vi "FH 55.vi"() -> ()   [LabVIEW 2014, in "FH 55.lvlib"]
uses:
  FH 55.lvlib
  TypeDef/VisaCluster.ctl
  TypeDef/command.ctl
  TypeDef/Unit.ctl
  TypeDef/Range.ctl
  TypeDef/Temp_Unit.ctl
  TypeDef/Max.ctl
  TypeDef/Unit2.ctl
  TypeDef/Display.ctl
  TypeDef/Value_String.ctl
panel:
  in  "Control":T6 {"Lower"."Numeric" format="%#_4f"; "Set_Rel"."Numeric" format="%#_4f"; "UPPER"."Numeric" format="%#_4f"}
  in  "Array":string[](array[string])
  out "measured values":string
  in  "measured values":cluster{"Numeric":i32, "OK Button":bool}
  out "FH 55 Gauss-/Teslameter":T7
  in  "Stop":bool
  in  "OK":bool
  out "Busy":bool
  in  "Cluster":T8
  in  "Init":bool
  in  "Local":bool
  in  "Reset":bool
  in  "Zero":bool
  out "time current":u32
  out "loop 2":i32
  out "loop 1":i32
  out "error out":errorcluster
  in  "error in (no error)":errorcluster
  out "VisaCluster":T9
  in  "VisaCluster":T9={"VISA Resource Name"="COM1"}
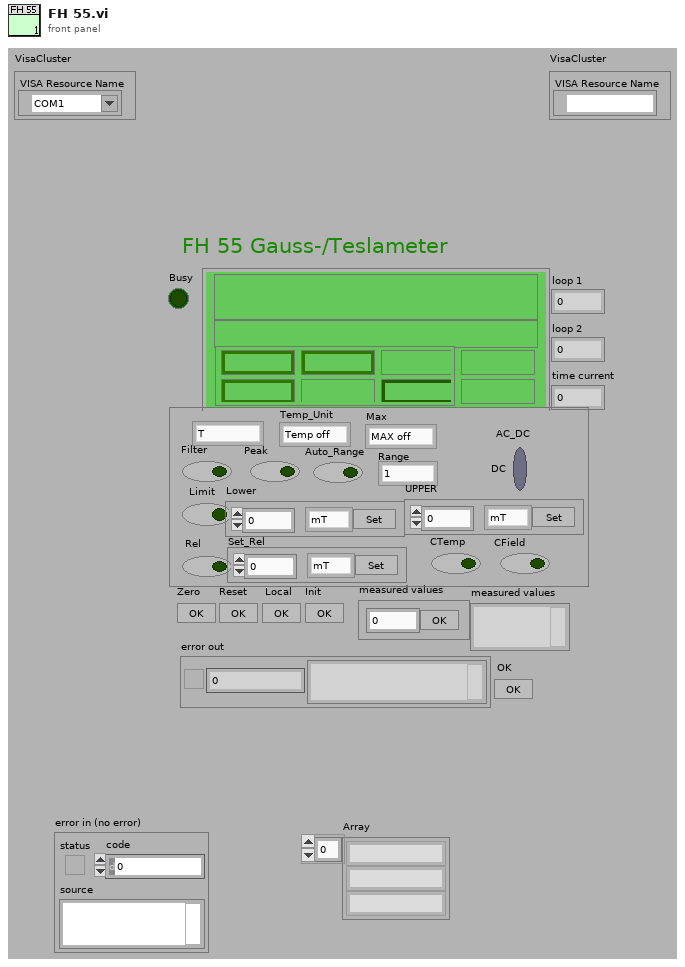
[diagram p1: front panel]
types:
  T1 = typedef "FH 55.lvlib/Range.ctl" = enum16{"1", "2", "3", "4", "5", "6", "7"}
  T2 = typedef "FH 55.lvlib/Unit2.ctl" = enum16{"mT", "G", "kA/m"}
  T3 = typedef "FH 55.lvlib/Unit.ctl" = enum16{"T", "G", "A/m"}
  T4 = typedef "FH 55.lvlib/Temp_Unit.ctl" = enum16{"Temp off", "Celsius", "Fahrenheit"}
  T5 = typedef "FH 55.lvlib/Max.ctl" = enum16{"MAX off", "Show MAX", "MAX/MIN"}
  T6 = cluster{" Peak":bool, " Limit":bool, " Filter":bool, " Auto_Range":bool, " Rel":bool, "AC_DC ":bool, "Range":T1, " CField":bool, " CTemp":bool, "UPPER":cluster{"Numeric":dbl, "Cancel Button":bool, "Unit":T2}, "Set_Rel":cluster{"Numeric":dbl, "Cancel Button":bool, "Unit":T2}, "Unit":T3, "Temp_Unit":T4, "Max":T5, "Lower":cluster{"Numeric":dbl, "Cancel Button":bool, "Unit":T2}}
  T7 = typedef "FH 55.lvlib/Display.ctl" = cluster{"current value":string, "Limit":string, "Remote":string, "function ":string, "Cluster":cluster{"AC/DC":string, "Auto":string, "Filter":string, "Range":string, "Rel":string, "Peak":string}}
  T8 = typedef "FH 55.lvlib/command.ctl" = cluster{"String":string, "Boolean":bool, "Unit":T3, "Range":T1, "Temp_Unit":T4, "Max":T5, "Numeric":i32, "Set_lower":cluster{"Numeric":i64, "Cancel Button":bool, "Unit":T2}}
  T9 = typedef "FH 55.lvlib/VisaCluster.ctl" = cluster{"VISA Resource Name":refnum<visa-resource-name>}
  T10 = cluster{"Peak":bool, "Limit":bool, "Filter":bool, "Auto_Range":bool, "Rel":bool, "AC_DC":bool, "Range":T1, "CField":bool, "CTemp":bool, "UPPER":cluster{"Numeric":dbl, "Cancel Button":bool, "Unit":T2}, "Set_Rel":cluster{"Numeric":dbl, "Cancel Button":bool, "Unit":T2}, "Unit":T3, "Temp_Unit":T4, "Max":T5, "Lower":cluster{"Numeric":dbl, "Cancel Button":bool, "Unit":T2}}
  T11 = typedef "FH 55.lvlib/Value_String.ctl" = cluster{"Numeric":dbl, "String":string}
  T12 = cluster{"current value":string, "Temperature":string, "Limit":string, "function":string, "Cluster":cluster{"AC/DC":string, "Auto":string, "Filter":string, "Range":string, "Rel":string, "Peak":string}}
  T13 = cluster{"AC/DC":string, "Auto":string, "Filter":string, "Range":string, "Rel":string, "Peak":string}
  T14 = typedef "Semaphore RefNum" = refnum<k1>
  T15 = cluster{"Numeric":i64, "Cancel Button":bool, "Unit":T2}
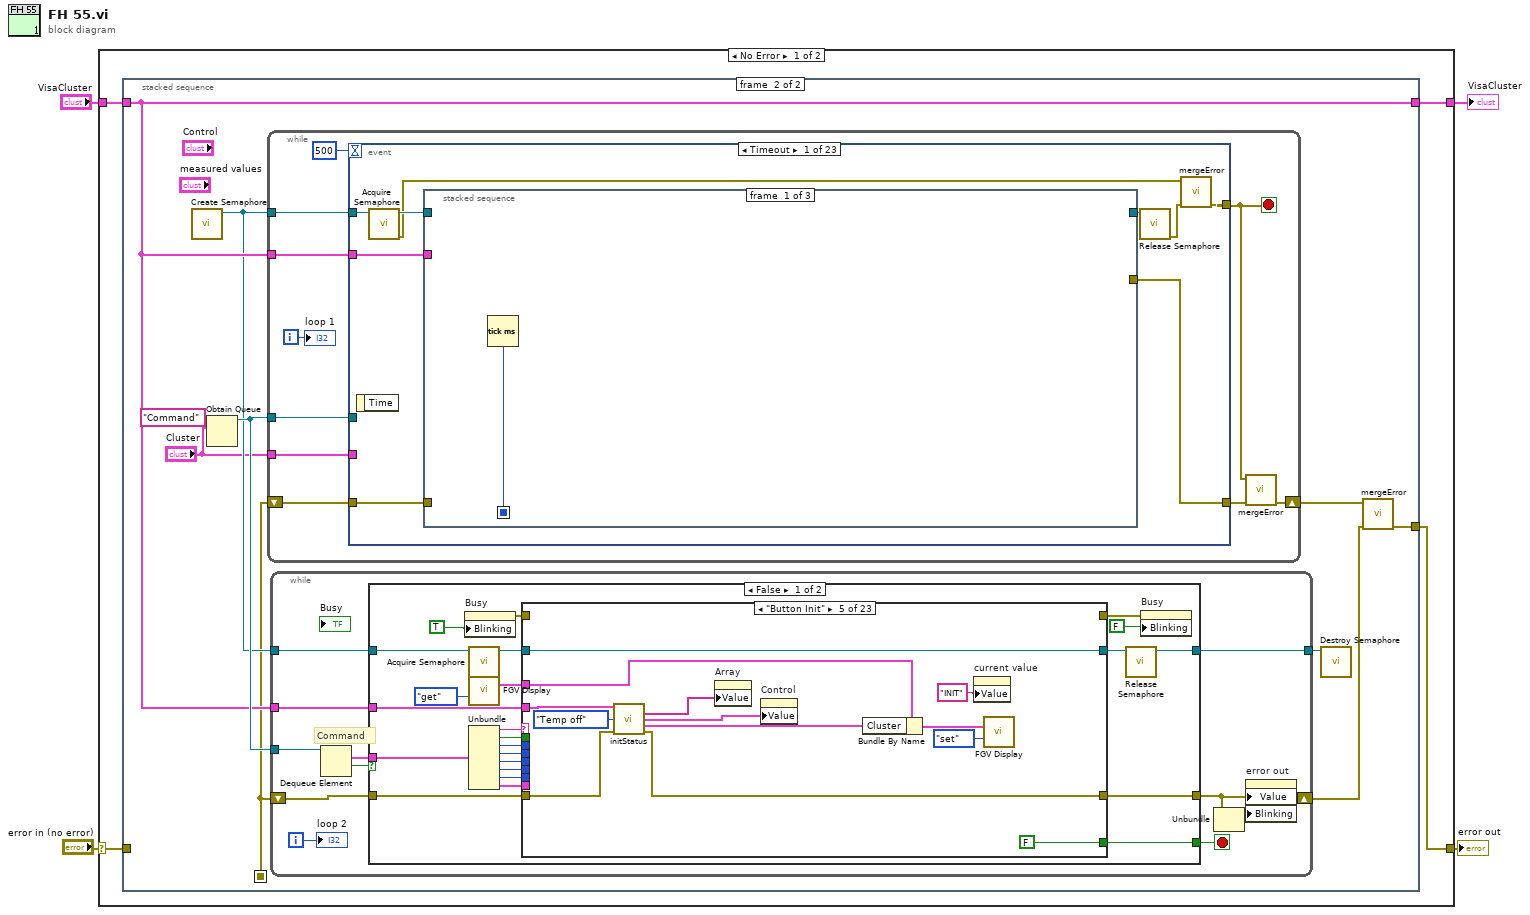
[diagram p0: block diagram]
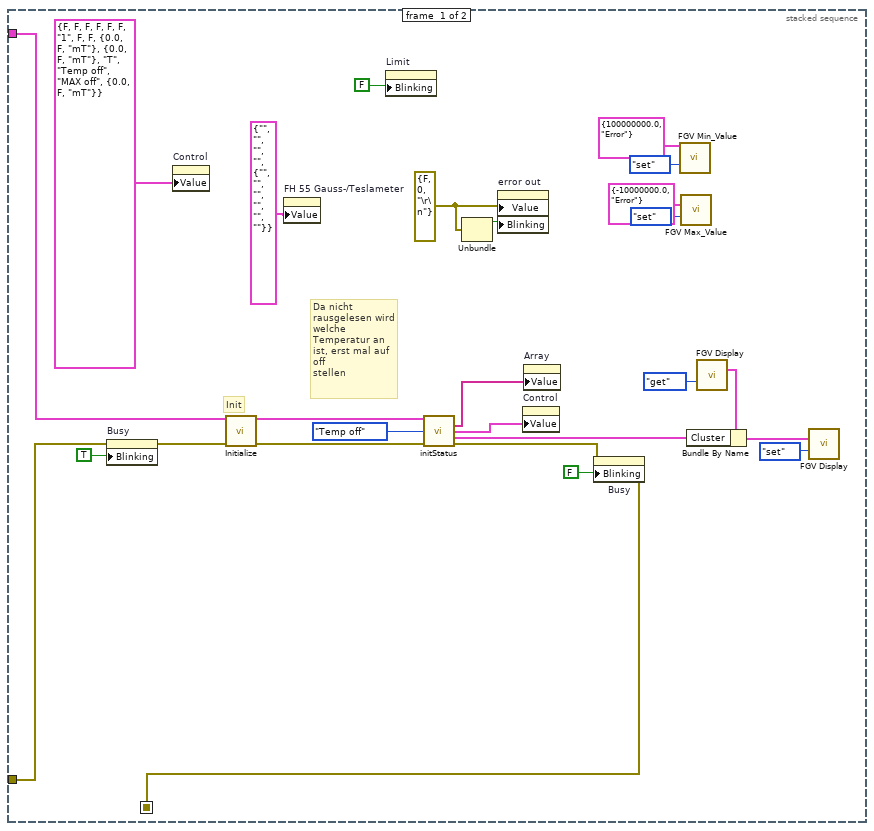
[diagram p2: hidden frame]
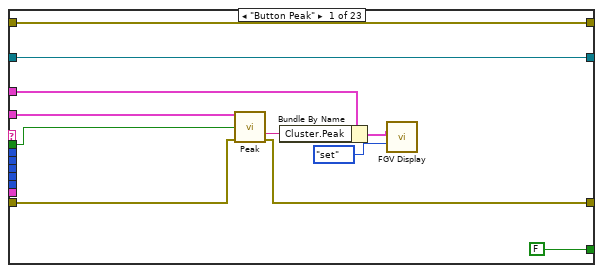
[diagram p3: hidden frame]
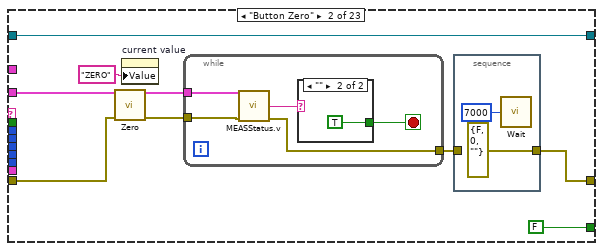
[diagram p4: hidden frame]
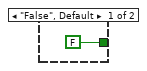
[diagram p5: hidden frame]
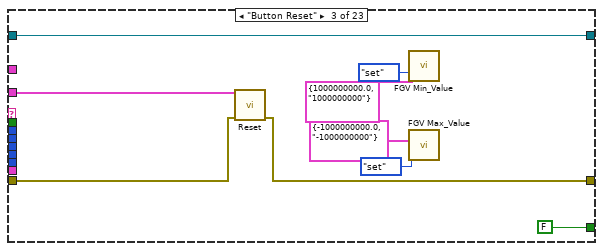
[diagram p6: hidden frame]
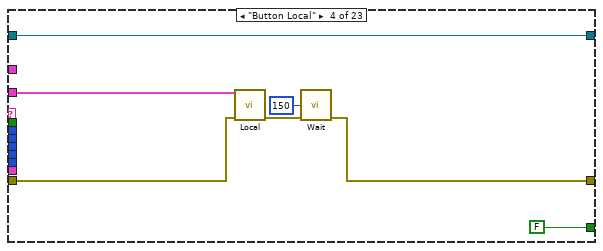
[diagram p7: hidden frame]
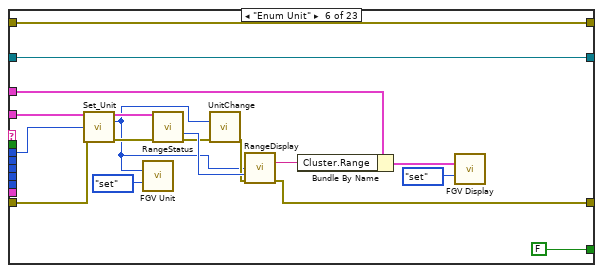
[diagram p8: hidden frame]
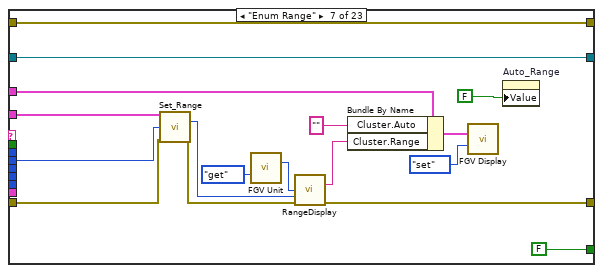
[diagram p9: hidden frame]
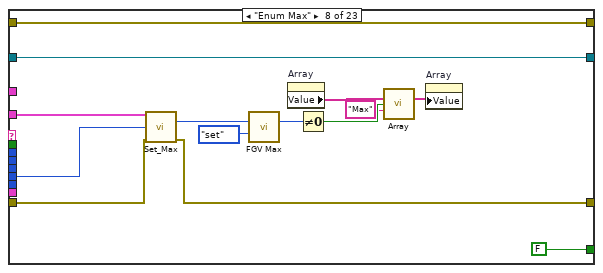
[diagram p10: hidden frame]
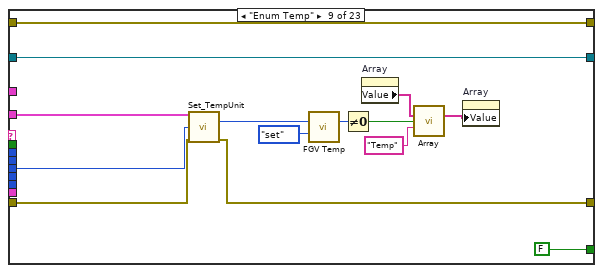
[diagram p11: hidden frame]
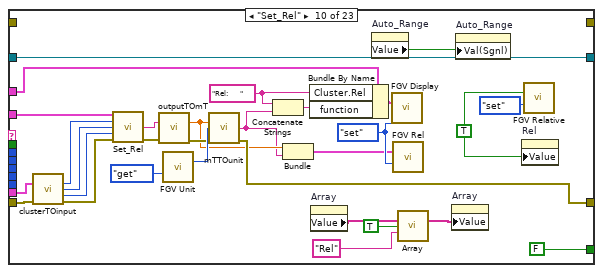
[diagram p12: hidden frame]
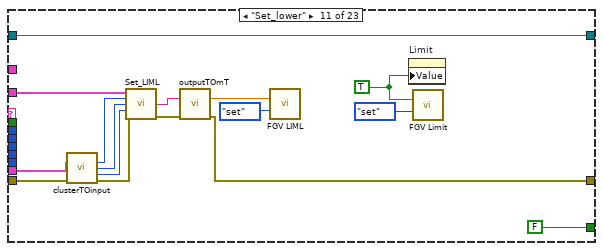
[diagram p13: hidden frame]
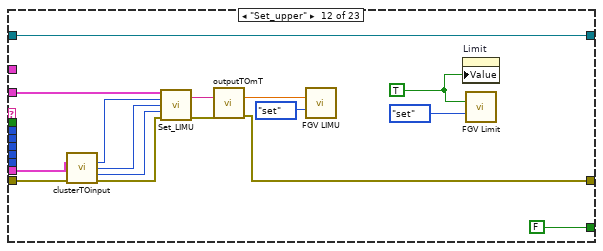
[diagram p14: hidden frame]
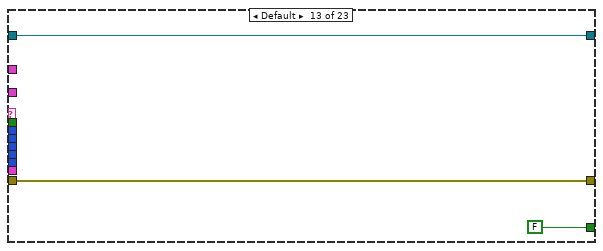
[diagram p15: hidden frame]
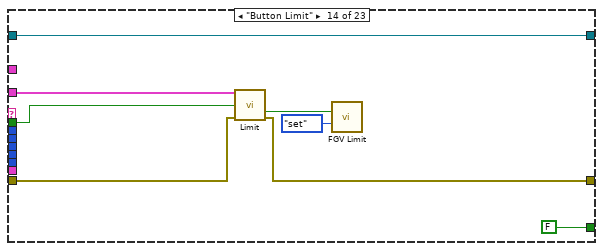
[diagram p16: hidden frame]
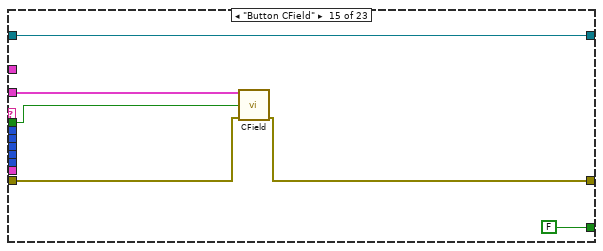
[diagram p17: hidden frame]
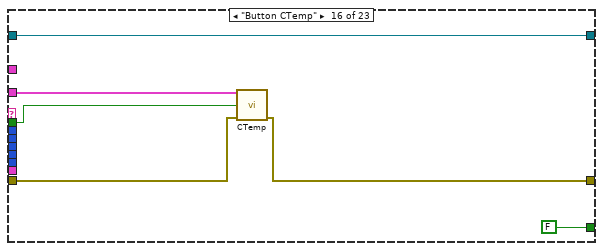
[diagram p18: hidden frame]
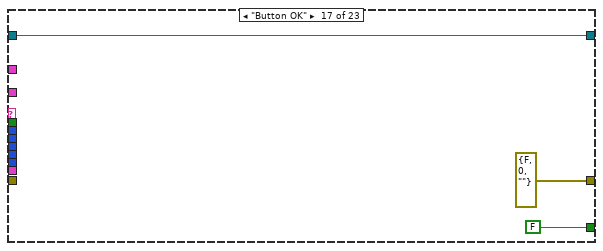
[diagram p19: hidden frame]
diagram:
  n1 = case shown="No Error" "error in (no error)" {
    selector: "error in (no error)" -> [w7 w591]
    tunnel: "VisaCluster" -> [w8 w592]
    tunnel: [w6 w592] -> w3
    tunnel: [w5 w591] -> w1
    frame No Error {
      n2 = stacked-sequence {
        seq-local: [w13 _] -> [_ w35]
        tunnel: w8 -> [w34 w42]
        tunnel: w7 -> [w22 _]
        tunnel: [_ w42] -> w6
        tunnel: [_ w39] -> w5
        frame #0 {
          w16 = errorcluster {"status"=FALSE, "code"=0, "source"="\r\n"} ("error out")
          # "Init"
          # "Da nicht rausgelesen wird welche \nTemperatur an ist, erst mal auf off \nstellen"
          n3 = property on="Busy" class="Bool (strict)"(error in=w22, "Blinking"=TRUE) -> (error out=w21:errorcluster)  [unwired: 1 in, 1 out]
          n4 = property on="Control" class="Clust (strict)"("Value"=T10 {"Peak"=FALSE, "Limit"=FALSE, "Filter"=FALSE, "Auto_Range"=FALSE, "Rel"=FALSE, "AC_DC"=FALSE, "Range"=enum."1", "CField"=FALSE, "CTemp"=FALSE, "UPPER"={"Numeric"=0.0, "Cancel Button"=FALSE, "Unit"=enum."mT"}, "Set_Rel"={"Numeric"=0.0, "Cancel Button"=FALSE, "Unit"=enum."mT"}, "Unit"=enum."T", "Temp_Unit"=enum."Temp off", "Max"=enum."MAX off", "Lower"={"Numeric"=0.0, "Cancel Button"=FALSE, "Unit"=enum."mT"}} ("Control")) -> ()  [unwired: 2 in, 2 out]
          n5 = call "Initialize.vi"("VisaCluster"=w34, "error in (no error)"=w21) -> ("VisaCluster"=w31:T9, "error out"=w30:errorcluster)  [unwired: 12 in]
          n6 = property on="FH 55 Gauss-/Teslameter" class="Clust (strict)"("Value"=T12 {"current value"="", "Temperature"="", "Limit"="", "function"="", "Cluster"={"AC/DC"="", "Auto"="", "Filter"="", "Range"="", "Rel"="", "Peak"=""}}) -> ()  [unwired: 2 in, 2 out]
          n7 = property on="Limit" class="Str"("Blinking"=FALSE) -> ()  [unwired: 2 in, 2 out]
          n8 = call "initStatus.vi"("VisaCluster"=w31, "Temp_Unit"=Temp_Unit."Temp off", "error in (no error)"=w30) -> ("Array"=w9:string[], "Control"=w10:T6, "Display"=w27:T13, "error out"=w24:errorcluster)  [unwired: 8 in, 1 out]
          n9 = Unbundle(w16) -> ("status"=w15:bool)  [unwired: 2 out]
          n10 = property on="error out" class="Clust (strict)"("Value"=w16, "Blinking"=w15) -> ()  [unwired: 2 in, 2 out]
          n11 = property on="Control" class="Clust (strict)"("Value"=w10) -> ()  [unwired: 2 in, 2 out]
          n12 = property on="Array" class="Arr (strict)"("Value"=w9) -> ()  [unwired: 2 in, 2 out]
          n13 = property on="Busy" class="Bool (strict)"(error in=w24, "Blinking"=FALSE) -> (error out=w13:errorcluster)  [unwired: 1 in, 1 out]
          n14 = call "FGV Min_Value.vi"("Extrem_Value"=T11 {"Numeric"=100000000.0, "String"="Error"}, "action"=enum16{"set", "get"}."set") -> ()  [unwired: 13 in, 1 out]
          n15 = call "FGV Max_Value.vi"("Extrem_Value"=T11 {"Numeric"=-10000000.0, "String"="Error"}, "action"=enum16{"set", "get"}."set") -> ()  [unwired: 13 in, 1 out]
          n16 = call "FGV Display.vi"("action"=enum16{"set", "get"}."get") -> ("FH 55 Gauss-/Teslameter 2"=w28:T7)  [unwired: 14 in]
          n17 = Bundle By Name(cluster=w28, "Cluster"=w27) -> (w26:T7)
          n18 = call "FGV Display.vi"("FH 55 Gauss-/Teslameter"=w26, "action"=enum16{"set", "get"}."set") -> ()  [unwired: 13 in, 1 out]
        }
        frame #1 {
          n19 = call <vilib>:"Create Semaphore.vi"() -> ("semaphore"=w41:T14)  [unwired: 5 in, 2 out]
          n20 = Obtain Queue(name (unnamed)="Command", element data type="Cluster") -> (queue out=w43:refnum<queue>)  [unwired: 3 in, 2 out]
          n21 = while {
            tunnel: w42 -> [w378]
            tunnel: w43 -> [w376]
            tunnel: "Cluster" -> [w375]
            tunnel: w41 -> [w374]
            shift-right: [w372] -> w36
            shift-left: w35 -> [w370]
            i -> [w369]
            stop <- w371 stop-if-true
            n22 = event shown="[0] Timeout" {
              selector: _ -> [_ _ _ _ _ _ _ _ _ _ _ _ _ _ _ _ _ _ _ _ _ _ _]
              dyn-events: _ -> [_ _ _ _ _ _ _ _ _ _ _ _ _ _ _ _ _ _ _ _ _ _ _]
              timeout: 500 -> [_ _ _ _ _ _ _ _ _ _ _ _ _ _ _ _ _ _ _ _ _ _ _]
              tunnel: w378 -> [w387 _ _ _ _ _ _ _ _ _ _ _ _ _ _ _ _ _ _ _ _ _ _]
              tunnel: w376 -> [_ w451 w457 w465 w475 w485 w495 w501 w508 w514 w520 w526 w532 w538 w544 w549 w554 w559 w564 w570 w576 w582 w588]
              tunnel: w375 -> [_ w452 w458 w464 w469 w480 w491 w500 w507 w513 w519 w525 w531 w537 w543 w548 w553 w558 w563 w569 w575 w581 w587]
              tunnel: w374 -> [w386 _ _ _ _ _ _ _ _ _ _ _ _ _ _ _ _ _ _ _ _ _ _]
              tunnel: [w382 _ _ _ _ _ _ _ _ _ _ _ _ _ _ _ _ _ _ _ _ _ _] -> w371
              tunnel: [w383 w450 w456 w463 w474 w484 w494 w499 w506 w512 w518 w524 w530 w536 w542 w547 w552 w557 w562 w568 w574 w580 w586] -> w373
              tunnel: w370 -> [w379 w450 w456 w463 w474 w484 w494 w499 w506 w512 w518 w524 w530 w536 w542 w547 w552 w557 w562 w568 w574 w580 w586]
              event Timeout {
                n23 = event-data() -> ()  [unwired: 1 in, 1 out]
                n24 = call <vilib>:"Acquire Semaphore.vi"("semaphore"=w386) -> ("error out"=w380:errorcluster, "semaphore out"=w385:T14)  [unwired: 4 in, 1 out]
                n25 = stacked-sequence {
                  seq-local: [w388 _ _] -> [_ _ w448]
                  tunnel: w387 -> [_ w417 _]
                  tunnel: w385 -> [_ w411 _]
                  tunnel: [_ w411 _] -> w384
                  tunnel: [_ w407 _] -> w383
                  tunnel: w379 -> [_ w404 _]
                  frame #0 {
                    n26 = Tick Count (ms)() -> (millisecond timer value=w388:u32)
                  }
                  frame #1 {
                    w391 = enum16{"set", "get"}."get" ("action")
                    n27 = call "FGV Max.vi"("action"=enum16{"set", "get"}."get") -> ("Max 2"=w400:T5)  [unwired: 14 in]
                    n28 = case shown="\"Show MAX\"" w400 {
                      tunnel: w417 -> [w427 w433 w439]
                      tunnel: [w426 w432 w438] -> w414
                      tunnel: w404 -> [w425 w431 w437]
                      tunnel: [w424 w430 w436] -> w403
                      tunnel: [w423 w429 w435] -> w401
                      frame "Show MAX" {
                        n29 = call "MEASStatus.v.vi"("VisaCluster"=w427, "Time (150) ms"=u32 200, "error in (no error)"=w425) -> ("VisaCluster"=w426:T9, "Answer"=w423:string, "error out"=w424:errorcluster)  [unwired: 10 in]
                      }
                      frame "MAX/MIN" {
                        n30 = call "MEASStatus.v.vi"("VisaCluster"=w433, "Time (150) ms"=u32 200, "error in (no error)"=w431) -> ("VisaCluster"=w432:T9, "Answer"=w429:string, "error out"=w430:errorcluster)  [unwired: 10 in]
                      }
                      frame "MAX off" {
                        n31 = call "MEASStatus.v.vi"("VisaCluster"=w439, "Time (150) ms"=u32 150, "error in (no error)"=w437) -> ("VisaCluster"=w438:T9, "Answer"=w435:string, "error out"=w436:errorcluster)  [unwired: 10 in]
                      }
                    }
                    n32 = call "FGV Limit.vi"("action"=enum16{"set", "get"}."get") -> ("Limit"=w408:bool)  [unwired: 14 in]
                    n33 = call "LimitFunktion.vi"("String"=w401, "Boolean"=w408) -> ("Answer"=w409:string)  [unwired: 12 in, 1 out]
                    n34 = call "MaxFunktion.vi"("VisaCluster"=w414, "Measurment"=w401, "Max"=w400, "error in (no error)"=w403) -> ("VisaCluster 2"=w413:T9, "Answer"=w395:string, "error out"=w402:errorcluster)  [unwired: 8 in, 1 out]
                    n35 = call "FGV Temp.vi"("action"=w391) -> ("Temp_Unit 2"=w412:T4)  [unwired: 14 in]
                    n36 = Index Array(array="Array", index=0) -> (element=w397:string)
                    n37 = case shown="True" w408 {
                      tunnel: w409 -> [_ w444]
                      frame False {
                        n38 = property on="Limit" class="Str"("Blinking"=FALSE) -> ()  [unwired: 2 in, 2 out]
                      }
                      frame True {
                        n39 = case shown="Default" w444 {
                          frame "OK" {
                            n40 = property on="Limit" class="Str"("Blinking"=FALSE) -> ()  [unwired: 2 in, 2 out]
                          }
                          frame Default {
                            n41 = property on="Limit" class="Str"("Blinking"=TRUE) -> ()  [unwired: 2 in, 2 out]
                          }
                        }
                      }
                    }
                    n42 = call "TempDisplay.vi"("VisaCluster"=w413, "Temp_Unit"=w412, "error in (no error)"=w402) -> ("Answer"=w396:string, "error out"=w393:errorcluster)  [unwired: 9 in, 2 out]
                    n43 = call "FGV Relative.vi"("action"=w391) -> ("Rel"=w389:bool)  [unwired: 14 in]
                    n44 = call "RelDisplay.vi"("Boolean"=w389, "error in (no error)"=w393) -> ("Answer"=w390:string, "error out"=w392:errorcluster)  [unwired: 11 in, 1 out]
                    n45 = case shown="Default" w397 {
                      tunnel: w396 -> [_ w419 _ _]
                      tunnel: w395 -> [w418 _ _ _]
                      tunnel: [w418 w419 w420 "" ("Answer")] -> w394
                      tunnel: w390 -> [_ _ w420 _]
                      frame "Max" {
                      }
                      frame "Temp" {
                      }
                      frame "Rel" {
                      }
                      frame Default {
                      }
                    }
                    n46 = case shown="Error" w392 {
                      selector: w392 -> [w440 w442]
                      tunnel: [w440 w442] -> w407
                      frame No Error {
                      }
                      frame Error {
                        n47 = property on="Stop" class="Bool (strict)"("Val(Sgnl)"=TRUE) -> ()  [unwired: 2 in, 2 out]
                      }
                    }
                    n48 = call "FGV Display.vi"("action"=enum16{"set", "get"}."get") -> ("FH 55 Gauss-/Teslameter 2"=w405:T7)  [unwired: 14 in]
                    n49 = Bundle By Name(cluster=w405, "function"=w394, "current value"=w401, "Limit"=w409) -> (→"FH 55 Gauss-/Teslameter":T7)
                  }
                  frame #2 {
                    n50 = Tick Count (ms)() -> (millisecond timer value=w449:u32)
                    n51 = Subtract(x=w449, y=w448) -> (x-y=→"time current":u32)
                  }
                }
                n52 = call <vilib>:"Release Semaphore.vi"("semaphore"=w384) -> ("error out"=w381:errorcluster)  [unwired: 5 in, 1 out]
                n53 = call "mergeError.vi"("error in (no error)"=w381, "error in (no error) 2"=w380) -> ("error out"=w382:errorcluster)  [unwired: 9 in]
              }
              event "OK": Value Change {
                n54 = event-data() -> ("NewVal"=w453:bool)  [unwired: 1 in]
                n55 = Bundle By Name(cluster=w452, "String"="Button OK" ("command"), "Boolean"=w453) -> (w454:T8)
                n56 = Enqueue Element(queue=w451, element=w454) -> ()  [unwired: 2 in, 3 out]
              }
              event "Stop": Value Change {
                n57 = event-data() -> ("NewVal"=w459:bool)  [unwired: 1 in]
                n58 = Bundle By Name(cluster=w458, "String"="Button Stop" ("command"), "Boolean"=w459) -> (w460:T8)
                n59 = Enqueue Element(queue=w457, element=w460) -> ()  [unwired: 2 in, 3 out]
              }
              event "Control.Peak": Value Change {
                n60 = event-data() -> ("NewVal"=w462:bool)  [unwired: 1 in]
                n61 = Bundle By Name(cluster=w464, "String"="Button Peak" ("command"), "Boolean"=w462) -> (w466:T8)
                n62 = Enqueue Element(queue=w465, element=w466) -> ()  [unwired: 2 in, 3 out]
              }
              event "Control.Set_Rel.Cancel Button": Value Change {
                n63 = event-data() -> ("OldVal"=w473:bool)  [unwired: 1 in]
                n64 = property on="Cancel Button" class="Bool (strict)"("Value"=w473) -> ()  [unwired: 2 in, 2 out]
                n65 = property on="Unit" class="Enum (strict)"() -> ("Value"=w471:T2)  [unwired: 2 in, 2 out]
                n66 = property on="Numeric" class="DigNum (strict)"() -> ("Value"=w472:dbl)  [unwired: 2 in, 2 out]
                n67 = Unbundle By Name(w469) -> ("Set_lower"=w468:T15)
                n68 = Bundle By Name(cluster=w468, "Numeric"=w472, "Unit"=w471) -> (w470:T15)
                n69 = Bundle By Name(cluster=w469, "String"="Set_Rel" ("command"), "Set_lower"=w470) -> (w476:T8)
                n70 = Enqueue Element(queue=w475, element=w476) -> ()  [unwired: 2 in, 3 out]
              }
              event "Control.Lower.Cancel Button": Value Change {
                n71 = event-data() -> ("OldVal"=w481:bool)  [unwired: 1 in]
                n72 = property on="Cancel Button" class="Bool (strict)"("Value"=w481) -> ()  [unwired: 2 in, 2 out]
                n73 = property on="Numeric" class="DigNum (strict)"() -> ("Value"=w483:dbl)  [unwired: 2 in, 2 out]
                n74 = property on="Unit" class="Enum (strict)"() -> ("Value"=w478:T2)  [unwired: 2 in, 2 out]
                n75 = Unbundle By Name(w480) -> ("Set_lower"=w479:T15)
                n76 = Bundle By Name(cluster=w479, "Numeric"=w483, "Unit"=w478) -> (w482:T15)
                n77 = Bundle By Name(cluster=w480, "String"="Set_lower" ("command"), "Set_lower"=w482) -> (w486:T8)
                n78 = Enqueue Element(queue=w485, element=w486) -> ()  [unwired: 2 in, 3 out]
              }
              event "Control.UPPER.Cancel Button": Value Change {
                n79 = event-data() -> ("OldVal"=w492:bool)  [unwired: 1 in]
                n80 = property on="Cancel Button" class="Bool (strict)"("Value"=w492) -> ()  [unwired: 2 in, 2 out]
                n81 = Unbundle By Name(w491) -> ("Set_lower"=w490:T15)
                n82 = property on="Numeric" class="DigNum (strict)"() -> ("Value"=w493:dbl)  [unwired: 2 in, 2 out]
                n83 = property on="Unit" class="Enum (strict)"() -> ("Value"=w489:T2)  [unwired: 2 in, 2 out]
                n84 = Bundle By Name(cluster=w490, "Numeric"=w493, "Unit"=w489) -> (w488:T15)
                n85 = Bundle By Name(cluster=w491, "String"="Set_upper" ("command"), "Set_lower"=w488) -> (w496:T8)
                n86 = Enqueue Element(queue=w495, element=w496) -> ()  [unwired: 2 in, 3 out]
              }
              event "Control.Limit": Value Change {
                n87 = event-data() -> ("NewVal"=w498:bool)  [unwired: 1 in]
                n88 = Bundle By Name(cluster=w500, "String"="Button Limit" ("command"), "Boolean"=w498) -> (w502:T8)
                n89 = Enqueue Element(queue=w501, element=w502) -> ()  [unwired: 2 in, 3 out]
              }
              event "measured values.OK Button": Value Change {
                n90 = event-data() -> ("OldVal"=w505:bool)  [unwired: 1 in]
                n91 = property on="OK Button" class="Bool (strict)"("Value"=w505) -> ()  [unwired: 2 in, 2 out]
                n92 = property on="Numeric" class="DigNum (strict)"() -> ("Value"=w504:i32)  [unwired: 2 in, 2 out]
                n93 = Bundle By Name(cluster=w507, "String"="Button Messwerte" ("command"), "Numeric"=w504) -> (w509:T8)
                n94 = Enqueue Element(queue=w508, element=w509) -> ()  [unwired: 2 in, 3 out]
              }
              event "Control.Filter": Value Change {
                n95 = event-data() -> ("NewVal"=w511:bool)  [unwired: 1 in]
                n96 = Bundle By Name(cluster=w513, "String"="Button Filter" ("command"), "Boolean"=w511) -> (w515:T8)
                n97 = Enqueue Element(queue=w514, element=w515) -> ()  [unwired: 2 in, 3 out]
              }
              event "Control.Auto_Range": Value Change {
                n98 = event-data() -> ("NewVal"=w517:bool)  [unwired: 1 in]
                n99 = Bundle By Name(cluster=w519, "String"="Button Auto_Range" ("command"), "Boolean"=w517) -> (w521:T8)
                n100 = Enqueue Element(queue=w520, element=w521) -> ()  [unwired: 2 in, 3 out]
              }
              event "Control.Rel": Value Change {
                n101 = event-data() -> ("NewVal"=w523:bool)  [unwired: 1 in]
                n102 = Bundle By Name(cluster=w525, "String"="Button Rel" ("command"), "Boolean"=w523) -> (w527:T8)
                n103 = Enqueue Element(queue=w526, element=w527) -> ()  [unwired: 2 in, 3 out]
              }
              event "Control.CField": Value Change {
                n104 = event-data() -> ("NewVal"=w529:bool)  [unwired: 1 in]
                n105 = Bundle By Name(cluster=w531, "String"="Button CField" ("command"), "Boolean"=w529) -> (w533:T8)
                n106 = Enqueue Element(queue=w532, element=w533) -> ()  [unwired: 2 in, 3 out]
              }
              event "Control.CTemp": Value Change {
                n107 = event-data() -> ("NewVal"=w535:bool)  [unwired: 1 in]
                n108 = Bundle By Name(cluster=w537, "String"="Button CTemp" ("command"), "Boolean"=w535) -> (w539:T8)
                n109 = Enqueue Element(queue=w538, element=w539) -> ()  [unwired: 2 in, 3 out]
              }
              event "Control.AC_DC": Value Change {
                n110 = event-data() -> ("NewVal"=w541:bool)  [unwired: 1 in]
                n111 = Bundle By Name(cluster=w543, "String"="Button AC_DC" ("command"), "Boolean"=w541) -> (w545:T8)
                n112 = Enqueue Element(queue=w544, element=w545) -> ()  [unwired: 2 in, 3 out]
              }
              event "Zero": Value Change {
                n113 = event-data() -> ()  [unwired: 1 in, 1 out]
                n114 = Bundle By Name(cluster=w548, "String"="Button Zero" ("command")) -> (w550:T8)
                n115 = Enqueue Element(queue=w549, element=w550) -> ()  [unwired: 2 in, 3 out]
              }
              event "Reset": Value Change {
                n116 = event-data() -> ()  [unwired: 1 in, 1 out]
                n117 = Bundle By Name(cluster=w553, "String"="Button Reset" ("command")) -> (w555:T8)
                n118 = Enqueue Element(queue=w554, element=w555) -> ()  [unwired: 2 in, 3 out]
              }
              event "Local": Value Change {
                n119 = event-data() -> ()  [unwired: 1 in, 1 out]
                n120 = Bundle By Name(cluster=w558, "String"="Button Local" ("command")) -> (w560:T8)
                n121 = Enqueue Element(queue=w559, element=w560) -> ()  [unwired: 2 in, 3 out]
              }
              event "Init": Value Change {
                n122 = event-data() -> ()  [unwired: 1 in, 1 out]
                n123 = Bundle By Name(cluster=w563, "String"="Button Init" ("command")) -> (w565:T8)
                n124 = Enqueue Element(queue=w564, element=w565) -> ()  [unwired: 2 in, 3 out]
              }
              event Value Change {
                n125 = event-data() -> ("NewVal"=w567:T3)  [unwired: 1 in]
                n126 = Bundle By Name(cluster=w569, "String"="Enum Unit" ("command"), "Unit"=w567) -> (w571:T8)
                n127 = Enqueue Element(queue=w570, element=w571) -> ()  [unwired: 2 in, 3 out]
              }
              event Value Change {
                n128 = event-data() -> ("NewVal"=w573:T1)  [unwired: 1 in]
                n129 = Bundle By Name(cluster=w575, "String"="Enum Range" ("command"), "Range"=w573) -> (w577:T8)
                n130 = Enqueue Element(queue=w576, element=w577) -> ()  [unwired: 2 in, 3 out]
              }
              event Value Change {
                n131 = event-data() -> ("NewVal"=w579:T5)  [unwired: 1 in, 5 out]
                n132 = Bundle By Name(cluster=w581, "String"="Enum Max" ("command"), "Max"=w579) -> (w583:T8)
                n133 = Enqueue Element(queue=w582, element=w583) -> ()  [unwired: 2 in, 3 out]
              }
              event Value Change {
                n134 = event-data() -> ("NewVal"=w585:T4)  [unwired: 1 in]
                n135 = Bundle By Name(cluster=w587, "String"="Enum Temp" ("command"), "Temp_Unit"=w585) -> (w589:T8)
                n136 = Enqueue Element(queue=w588, element=w589) -> ()  [unwired: 2 in, 3 out]
              }
            }
            n137 = call "mergeError.vi"("error in (no error)"=w373, "error in (no error) 2"=w371) -> ("error out"=w372:errorcluster)  [unwired: 9 in]
            "loop 1" <- w369
          }
          n138 = while {
            tunnel: w43 -> [w55]
            tunnel: w42 -> [w52]
            tunnel: w41 -> [w50]
            tunnel: [w49] -> w40
            shift-right: [w46] -> w37
            shift-left: w35 -> [w48]
            i -> [w51]
            stop <- w47 stop-if-true
            # "Command"
            n139 = Dequeue Element(queue=w55) -> (element=w53:T8, timed out?=w54:bool)  [unwired: 2 in, 2 out]
            n140 = case shown="False" w54 {
              tunnel: w53 -> [w78 _]
              tunnel: w52 -> [w76 _]
              tunnel: w50 -> [w74 w368]
              tunnel: [w71 w368] -> w49
              tunnel: w48 -> [w70 w367]
              tunnel: [w69 w367] -> w46
              tunnel: [w58 FALSE ("Boolean")] -> w47
              frame False {
                n141 = property on="Busy" class="Bool (strict)"("Blinking"=TRUE) -> (error out=w61:errorcluster)  [unwired: 2 in, 1 out]
                n142 = call <vilib>:"Acquire Semaphore.vi"("semaphore"=w74) -> ("semaphore out"=w73:T14)  [unwired: 4 in, 2 out]
                n143 = call "FGV Display.vi"("action"=enum16{"set", "get"}."get") -> ("FH 55 Gauss-/Teslameter 2"=w57:T7)  [unwired: 14 in]
                n144 = Unbundle(w78) -> ("String"=w75:string, "Boolean"=w77:bool, "Unit"=w67:T3, "Range"=w66:T1, "Temp_Unit"=w64:T4, "Max"=w65:T5, "Numeric"=w63:i32, "Set_lower"=w56:T15)
                n145 = case shown="\"Button Init\"" w75 {
                  tunnel: w77 -> [w89 _ _ _ _ _ _ _ _ _ _ _ _ w270 w273 w280 _ w286 w298 _ w331 w354 w364]
                  tunnel: w76 -> [w88 w98 w116 w123 w134 w152 w169 w182 w195 w226 w242 w258 _ w269 w275 w281 _ _ w297 w308 w330 w353 w365]
                  tunnel: w73 -> [w87 w97 w115 w122 w136 w154 w171 w184 w197 w227 w243 w259 w262 w268 w276 w282 w285 w288 w296 w310 w329 w352 w363]
                  tunnel: [w87 w97 w115 w122 w136 w154 w171 w184 w197 w227 w243 w259 w262 w268 w276 w282 w285 w288 w296 w310 w329 w352 w363] -> w72
                  tunnel: w70 -> [w86 w96 w114 w121 w133 w153 w170 w183 w196 w219 w234 w250 w261 w267 w274 w279 _ w287 w295 w307 w328 w351 w362]
                  tunnel: [w85 w91 w113 w118 w127 w145 w165 w180 w193 w211 w231 w247 w261 w266 w272 w278 errorcluster {"status"=FALSE, "code"=0, "source"=""} ("error out") w287 w294 w303 w314 w350 w361] -> w69
                  tunnel: w67 -> [_ _ _ _ _ w151 _ _ _ _ _ _ _ _ _ _ _ _ _ _ _ _ _]
                  tunnel: w66 -> [_ _ _ _ _ _ w168 _ _ _ _ _ _ _ _ _ _ _ _ _ _ _ _]
                  tunnel: w65 -> [_ _ _ _ _ _ _ w181 _ _ _ _ _ _ _ _ _ _ _ _ _ _ _]
                  tunnel: w64 -> [_ _ _ _ _ _ _ _ w192 _ _ _ _ _ _ _ _ _ _ _ _ _ _]
                  tunnel: w63 -> [_ _ _ _ _ _ _ _ _ _ _ _ _ _ _ _ _ _ _ w302 _ _ _]
                  tunnel: w61 -> [w79 _ _ _ _ w140 w156 w177 w190 _ _ _ _ _ _ _ _ _ _ _ w319 w344 w355]
                  tunnel: [w79 _ _ _ _ w140 w156 w177 w190 _ _ _ _ _ _ _ _ _ _ _ w319 w344 w355] -> w60
                  tunnel: [FALSE ("Boolean") FALSE ("Boolean") FALSE ("Boolean") FALSE ("Boolean") FALSE ("Boolean") FALSE ("Boolean") FALSE ("Boolean") FALSE ("Boolean") FALSE ("Boolean") FALSE ("Boolean") FALSE ("Boolean") FALSE ("Boolean") FALSE ("Boolean") FALSE ("Boolean") FALSE ("Boolean") FALSE ("Boolean") FALSE ("Boolean") w286 FALSE ("Boolean") FALSE ("Boolean") FALSE ("Boolean") FALSE ("Boolean") FALSE ("Boolean")] -> w58
                  tunnel: w57 -> [w81 _ _ _ w131 w142 w158 _ _ w221 _ _ _ _ _ _ _ _ w290 _ w317 w346 w357]
                  tunnel: w56 -> [_ _ _ _ _ _ _ _ _ w205 w229 w245 _ _ _ _ _ _ _ _ _ _ _]
                  frame "Button Peak" {
                    n146 = call "Peak.vi"("VisaCluster"=w88, "Peak"=w89, "error in (no error)"=w86) -> ("Display"=w83:string, "error out"=w85:errorcluster)  [unwired: 8 in, 3 out]
                    n147 = Bundle By Name(cluster=w81, "Cluster.Peak"=w83) -> (w80:T7)
                    n148 = call "FGV Display.vi"("FH 55 Gauss-/Teslameter"=w80, "action"=enum16{"set", "get"}."set") -> ()  [unwired: 13 in, 1 out]
                  }
                  frame "Button Zero" {
                    n149 = call "Zero.vi"("VisaCluster"=w98, "error in (no error)"=w96) -> ("VisaCluster"=w94:T9, "error out"=w93:errorcluster)  [unwired: 11 in, 1 out]
                    n150 = property on="current value" class="Str"("Value"="ZERO") -> ()  [unwired: 2 in, 2 out]
                    n151 = while {
                      tunnel: w94 -> [w105]
                      tunnel: w93 -> [w102]
                      tunnel: [w101] -> w92
                      stop <- w103 stop-if-true
                      n152 = call "MEASStatus.v.vi"("VisaCluster"=w105, "error in (no error)"=w102) -> ("Answer"=w104:string, "error out"=w101:errorcluster)  [unwired: 11 in, 1 out]
                      n153 = case shown="\"\"" w104 {
                        tunnel: [FALSE TRUE] -> w103
                        frame "False", Default {
                        }
                        frame "" {
                        }
                      }
                    }
                    n154 = stacked-sequence {
                      tunnel: w92 -> [_]
                      tunnel: [errorcluster {"status"=FALSE, "code"=0, "source"=""} ("error out")] -> w91
                      frame #0 {
                        n155 = call "Wait.vi"("milliseconds to wait"=u32 7000) -> ()  [unwired: 14 in, 1 out]
                      }
                    }
                  }
                  frame "Button Reset" {
                    n156 = call "Reset.vi"("VisaCluster"=w116, "error in (no error)"=w114) -> ("error out"=w113:errorcluster)  [unwired: 11 in, 2 out]
                    n157 = call "FGV Min_Value.vi"("Extrem_Value"=T11 {"Numeric"=1000000000.0, "String"="1000000000"}, "action"=enum16{"set", "get"}."set") -> ()  [unwired: 13 in, 1 out]
                    n158 = call "FGV Max_Value.vi"("Extrem_Value"=T11 {"Numeric"=-1000000000.0, "String"="-1000000000"}, "action"=enum16{"set", "get"}."set") -> ()  [unwired: 13 in, 1 out]
                  }
                  frame "Button Local" {
                    n159 = call "Local.vi"("VisaCluster"=w123, "error in (no error)"=w121) -> ("error out"=w119:errorcluster)  [unwired: 11 in, 2 out]
                    n160 = call "Wait.vi"("milliseconds to wait"=u32 150, "error in (no error)"=w119) -> ("error out"=w118:errorcluster)  [unwired: 13 in]
                  }
                  frame "Button Init" {
                    n161 = call "initStatus.vi"("VisaCluster"=w134, "Temp_Unit"=Temp_Unit."Temp off", "error in (no error)"=w133) -> ("Array"=w125:string[], "Control"=w124:T6, "Display"=w130:T13, "error out"=w127:errorcluster)  [unwired: 8 in, 1 out]
                    n162 = property on="Array" class="Arr (strict)"("Value"=w125) -> ()  [unwired: 2 in, 2 out]
                    n163 = property on="Control" class="Clust (strict)"("Value"=w124) -> ()  [unwired: 2 in, 2 out]
                    n164 = Bundle By Name(cluster=w131, "Cluster"=w130) -> (w129:T7)
                    n165 = property on="current value" class="Str"("Value"="INIT") -> ()  [unwired: 2 in, 2 out]
                    n166 = call "FGV Display.vi"("FH 55 Gauss-/Teslameter"=w129, "action"=enum16{"set", "get"}."set") -> ()  [unwired: 13 in, 1 out]
                  }
                  frame "Enum Unit" {
                    n167 = call "Set_Unit.vi"("VisaCluster"=w152, "Unit"=w151, "error in (no error)"=w153) -> ("VisaCluster"=w150:T9, "Unit"=w137:T3, "error out"=w148:errorcluster)  [unwired: 9 in, 1 out]
                    n168 = call "FGV Unit.vi"("Unit"=w137, "action"=enum16{"set", "get"}."set") -> ()  [unwired: 13 in, 1 out]
                    n169 = call "RangeStatus.vi"("VisaCluster"=w150, "error in (no error)"=w148) -> ("Range"=w147:T1, "error out"=w139:errorcluster)  [unwired: 10 in, 2 out]
                    n170 = call "UnitChange.vi"("Unit"=w137, "error in (no error)"=w139) -> ("error out"=w138:errorcluster)  [unwired: 13 in]
                    n171 = call "RangeDisplay.vi"("Unit"=w137, "Range"=w147, "error in (no error)"=w138) -> ("Display"=w146:string, "error out"=w145:errorcluster)  [unwired: 10 in, 1 out]
                    n172 = Bundle By Name(cluster=w142, "Cluster.Range"=w146) -> (w141:T7)
                    n173 = call "FGV Display.vi"("FH 55 Gauss-/Teslameter"=w141, "action"=enum16{"set", "get"}."set") -> ()  [unwired: 13 in, 1 out]
                  }
                  frame "Enum Range" {
                    n174 = call "Set_Range.vi"("VisaCluster"=w169, "Range"=w168, "error in (no error)"=w170) -> ("Range"=w166:T1, "error out"=w162:errorcluster)  [unwired: 9 in, 2 out]
                    n175 = call "FGV Unit.vi"("action"=enum16{"set", "get"}."get") -> ("Unit"=w160:T3)  [unwired: 14 in]
                    n176 = call "RangeDisplay.vi"("Unit"=w160, "Range"=w166, "error in (no error)"=w162) -> ("Display"=w164:string, "error out"=w165:errorcluster)  [unwired: 10 in, 1 out]
                    n177 = Bundle By Name(cluster=w158, "Cluster.Auto"="" ("Auto"), "Cluster.Range"=w164) -> (w157:T7)
                    n178 = call "FGV Display.vi"("FH 55 Gauss-/Teslameter"=w157, "action"=enum16{"set", "get"}."set") -> ()  [unwired: 13 in, 1 out]
                    n179 = property on="Auto_Range" class="Bool (strict)"("Value"=FALSE ("Auto_\nRange")) -> ()  [unwired: 2 in, 2 out]
                  }
                  frame "Enum Max" {
                    n180 = call "Set_Max.vi"("VisaCluster"=w182, "Max"=w181, "error in (no error)"=w183) -> ("Max 2"=w174:T5, "error out"=w180:errorcluster)  [unwired: 9 in, 2 out]
                    n181 = call "FGV Max.vi"("Max"=w174, "action"=enum16{"set", "get"}."set") -> ()  [unwired: 13 in, 1 out]
                    n182 = property on="Array" class="Arr (strict)"() -> ("Value"=w176:string[])  [unwired: 2 in, 2 out]
                    n183 = Not Equal To 0?(x=w174) -> (x != 0?=w173:bool)
                    n184 = call "Array.vi"("Array"=w176, "Boolean"=w173, "String"="Max") -> ("Array"=w175:string[])  [unwired: 12 in]
                    n185 = property on="Array" class="Arr (strict)"("Value"=w175) -> ()  [unwired: 2 in, 2 out]
                  }
                  frame "Enum Temp" {
                    n186 = call "Set_TempUnit.vi"("VisaCluster"=w195, "Temp_Unit"=w192, "error in (no error)"=w196) -> ("Temp_Unit"=w187:T4, "error out"=w193:errorcluster)  [unwired: 9 in, 2 out]
                    n187 = call "FGV Temp.vi"("Temp_Unit"=w187, "action"=enum16{"set", "get"}."set") -> ()  [unwired: 13 in, 1 out]
                    n188 = Not Equal To 0?(x=w187) -> (x != 0?=w186:bool)
                    n189 = property on="Array" class="Arr (strict)"() -> ("Value"=w189:string[])  [unwired: 2 in, 2 out]
                    n190 = call "Array.vi"("Array"=w189, "Boolean"=w186, "String"="Temp" ("element")) -> ("Array"=w188:string[])  [unwired: 12 in]
                    n191 = property on="Array" class="Arr (strict)"("Value"=w188) -> ()  [unwired: 2 in, 2 out]
                  }
                  frame "Set_Rel" {
                    w212 = enum16{"set", "get"}."set" ("action")
                    w199 = "Rel:      " ("Rel")
                    w203 = TRUE ("Rel")
                    n192 = call "clusterTOinput.vi"("Set_Rel"=w205, "error in (no error)"=w219) -> ("Range"=w225:T1, "Numeric"=w224:i32, "Unit"=w223:T3, "error out"=w218:errorcluster)  [unwired: 10 in]
                    n193 = call "Set_Rel.vi"("VisaCluster"=w226, "Range"=w225, "Numeric"=w224, "Unit"=w223, "error in (no error)"=w218) -> ("Answer"=w216:string, "error out"=w217:errorcluster)  [unwired: 8 in, 1 out]
                    n194 = call "outputTOmT.vi"("Input"=w216, "error in (no error)"=w217) -> ("Numeric"=w202:dbl, "error out"=w213:errorcluster)  [unwired: 12 in]
                    n195 = call "FGV Unit.vi"("action"=enum16{"set", "get"}."get") -> ("Unit"=w214:T3)  [unwired: 14 in]
                    n196 = call "mTTOunit.vi"("Numeric"=w202, "Unit"=w214, "error in (no error)"=w213) -> ("Display"=w200:string, "error out"=w211:errorcluster)  [unwired: 10 in, 1 out]
                    n197 = Concatenate Strings(w199, w200) -> (w198:string)
                    n198 = Bundle("Numeric"=w202, "Display"=w200) -> (w201:cluster{"Numeric":dbl, "Display":string})  [unwired: 1 in]
                    n199 = Bundle By Name(cluster=w221, "Cluster.Rel"=w199, "function"=w198) -> (w220:T7)
                    n200 = property on="Array" class="Arr (strict)"() -> ("Value"=w209:string[])  [unwired: 2 in, 2 out]
                    n201 = property on="Auto_Range" class="Bool (strict)"() -> ("Value"=w204:bool)  [unwired: 2 in, 2 out]
                    n202 = call "FGV Display.vi"("FH 55 Gauss-/Teslameter"=w220, "action"=w212) -> ()  [unwired: 13 in, 1 out]
                    n203 = call "FGV Rel.vi"("Extrem_Value"=w201, "action"=w212) -> ()  [unwired: 12 in, 2 out]
                    n204 = call "Array.vi"("Array"=w209, "Boolean"=TRUE, "String"="Rel" ("element")) -> ("Array"=w206:string[])  [unwired: 12 in]
                    n205 = property on="Array" class="Arr (strict)"("Value"=w206) -> ()  [unwired: 2 in, 2 out]
                    n206 = property on="Auto_Range" class="Bool (strict)"("Val(Sgnl)"=w204) -> ()  [unwired: 2 in, 2 out]
                    n207 = property on="Rel" class="Bool (strict)"("Value"=w203) -> ()  [unwired: 2 in, 2 out]
                    n208 = call "FGV Relative.vi"("Rel"=w203, "action"=enum16{"set", "get"}."set") -> ()  [unwired: 13 in, 1 out]
                  }
                  frame "Set_lower" {
                    w228 = TRUE
                    n209 = call "clusterTOinput.vi"("Set_Rel"=w229, "error in (no error)"=w234) -> ("Range"=w241:T1, "Numeric"=w240:i32, "Unit"=w239:T3, "error out"=w233:errorcluster)  [unwired: 10 in]
                    n210 = call "Set_LIML.vi"("VisaCluster"=w242, "Range"=w241, "Ziffern"=w240, "Unit"=w239, "error in (no error)"=w233) -> ("Answer"=w237:string, "error out"=w232:errorcluster)  [unwired: 8 in, 1 out]
                    n211 = call "outputTOmT.vi"("Input"=w237, "error in (no error)"=w232) -> ("Numeric"=w236:dbl, "error out"=w231:errorcluster)  [unwired: 12 in]
                    n212 = call "FGV LIML.vi"("Numeric"=w236, "action"=enum16{"set", "get"}."set") -> ()  [unwired: 13 in, 1 out]
                    n213 = property on="Limit" class="Bool (strict)"("Value"=w228) -> ()  [unwired: 2 in, 2 out]
                    n214 = call "FGV Limit.vi"("Limit"=w228, "action"=enum16{"set", "get"}."set") -> ()  [unwired: 13 in, 1 out]
                  }
                  frame "Set_upper" {
                    w244 = TRUE
                    n215 = call "clusterTOinput.vi"("Set_Rel"=w245, "error in (no error)"=w250) -> ("Range"=w251:T1, "Numeric"=w252:i32, "Unit"=w257:T3, "error out"=w249:errorcluster)  [unwired: 10 in]
                    n216 = call "Set_LIMU.vi"("VisaCluster"=w258, "Range"=w251, "Ziffern"=w252, "Unit"=w257, "error in (no error)"=w249) -> ("Answer"=w255:string, "error out"=w248:errorcluster)  [unwired: 8 in, 1 out]
                    n217 = call "outputTOmT.vi"("Input"=w255, "error in (no error)"=w248) -> ("Numeric"=w254:dbl, "error out"=w247:errorcluster)  [unwired: 12 in]
                    n218 = call "FGV LIMU.vi"("Numeric"=w254, "action"=enum16{"set", "get"}."set") -> ()  [unwired: 13 in, 1 out]
                    n219 = property on="Limit" class="Bool (strict)"("Value"=w244) -> ()  [unwired: 2 in, 2 out]
                    n220 = call "FGV Limit.vi"("Limit"=w244, "action"=enum16{"set", "get"}."set") -> ()  [unwired: 13 in, 1 out]
                  }
                  frame Default {
                  }
                  frame "Button Limit" {
                    n221 = call "Limit.vi"("VisaCluster"=w269, "Limit"=w270, "error in (no error)"=w267) -> ("Limit"=w265:bool, "error out"=w266:errorcluster)  [unwired: 9 in, 2 out]
                    n222 = call "FGV Limit.vi"("Limit"=w265, "action"=enum16{"set", "get"}."set") -> ()  [unwired: 13 in, 1 out]
                  }
                  frame "Button CField" {
                    n223 = call "CField.vi"("VisaCluster"=w275, "CField"=w273, "error in (no error)"=w274) -> ("error out"=w272:errorcluster)  [unwired: 9 in, 3 out]
                  }
                  frame "Button CTemp" {
                    n224 = call "CTemp.vi"("VisaCluster"=w281, "CTemp"=w280, "error in (no error)"=w279) -> ("error out"=w278:errorcluster)  [unwired: 9 in, 3 out]
                  }
                  frame "Button OK" {
                  }
                  frame "Button Stop" {
                  }
                  frame "Button Filter" {
                    n225 = call "Filter.vi"("VisaCluster"=w297, "Filter"=w298, "error in (no error)"=w295) -> ("Display"=w292:string, "error out"=w294:errorcluster)  [unwired: 8 in, 3 out]
                    n226 = Bundle By Name(cluster=w290, "Cluster.Filter"=w292) -> (w289:T7)
                    n227 = call "FGV Display.vi"("FH 55 Gauss-/Teslameter"=w289, "action"=enum16{"set", "get"}."set") -> ()  [unwired: 13 in, 1 out]
                  }
                  frame "Button Messwerte" {
                    n228 = call "Set_NMeas.vi"("VisaCluster"=w308, "measured values"=w302, "error in (no error)"=w307) -> ("VisaCluster"=w305:T9, "error out"=w304:errorcluster)  [unwired: 10 in, 1 out]
                    n229 = call "Multi.vi"("VisaCluster"=w305, "Multi"=TRUE, "error in (no error)"=w304) -> ("Answer"=w301:string, "error out"=w303:errorcluster)  [unwired: 10 in, 1 out]
                    n230 = Match Pattern(string=w301, regular expression="MULTI 1\r\n") -> (after substring=→"measured values":string)  [unwired: 1 in, 3 out]
                  }
                  frame "Button Auto_Range" {
                    n231 = call "Auto_Range.vi"("VisaCluster"=w330, "Auto_Range"=w331, "error in (no error)"=w328) -> ("VisaCluster"=w313:T9, "Auto"=w315:bool, "Display"=w323:string, "error out"=w322:errorcluster)  [unwired: 8 in, 1 out]
                    n232 = case shown="True" w315 {
                      tunnel: [w333 w337] -> w324
                      tunnel: w322 -> [w333 w335]
                      tunnel: w313 -> [w332 w334]
                      tunnel: [w332 w334] -> w312
                      frame False {
                      }
                      frame True {
                        n233 = call "Wait.vi"("milliseconds to wait"=u32 2000, "error in (no error)"=w335) -> ("error out"=w337:errorcluster)  [unwired: 13 in]
                      }
                    }
                    n234 = call "FGV Unit.vi"("action"=enum16{"set", "get"}."get") -> ("Unit"=w320:T3)  [unwired: 14 in]
                    n235 = call "RangeStatus.vi"("VisaCluster"=w312, "error in (no error)"=w324) -> ("Range"=w311:T1, "error out"=w325:errorcluster)  [unwired: 10 in, 2 out]
                    n236 = call "RangeDisplay.vi"("Unit"=w320, "Range"=w311, "error in (no error)"=w325) -> ("Display"=w326:string, "error out"=w314:errorcluster)  [unwired: 10 in, 1 out]
                    n237 = property on="Range" class="Enum (strict)"("Value"=w311) -> ()  [unwired: 2 in, 2 out]
                    n238 = Bundle By Name(cluster=w317, "Cluster.Auto"=w323, "Cluster.Range"=w326) -> (w316:T7)
                    n239 = call "FGV Display.vi"("FH 55 Gauss-/Teslameter"=w316, "action"=enum16{"set", "get"}."set") -> ()  [unwired: 13 in, 1 out]
                  }
                  frame "Button Rel" {
                    n240 = call "Rel.vi"("VisaCluster"=w353, "Rel"=w354, "error in (no error)"=w351) -> ("Boolean"=w340:bool, "Display"=w349:string, "error out"=w350:errorcluster)  [unwired: 8 in, 2 out]
                    n241 = Bundle By Name(cluster=w346, "Cluster.Rel"=w349) -> (w345:T7)
                    n242 = call "FGV Relative.vi"("Rel"=w340, "action"=enum16{"set", "get"}."set") -> ()  [unwired: 13 in, 1 out]
                    n243 = property on="Array" class="Arr (strict)"() -> ("Value"=w341:string[])  [unwired: 2 in, 2 out]
                    n244 = call "FGV Display.vi"("FH 55 Gauss-/Teslameter"=w345, "action"=enum16{"set", "get"}."set") -> ()  [unwired: 13 in, 1 out]
                    n245 = call "Array.vi"("Array"=w341, "Boolean"=w340, "String"="Rel" ("element")) -> ("Array"=w342:string[])  [unwired: 12 in]
                    n246 = property on="Auto_Range" class="Bool (strict)"() -> ("Value"=w338:bool)  [unwired: 2 in, 2 out]
                    n247 = property on="Auto_Range" class="Bool (strict)"("Val(Sgnl)"=w338) -> ()  [unwired: 2 in, 2 out]
                    n248 = property on="Array" class="Arr (strict)"("Value"=w342) -> ()  [unwired: 2 in, 2 out]
                  }
                  frame "Button AC_DC" {
                    n249 = call "AC_DC.vi"("VisaCluster"=w365, "AC_DC"=w364, "error in (no error)"=w362) -> ("Display"=w359:string, "error out"=w361:errorcluster)  [unwired: 8 in, 3 out]
                    n250 = Bundle By Name(cluster=w357, "Cluster.AC/DC"=w359) -> (w356:T7)
                    n251 = call "FGV Display.vi"("FH 55 Gauss-/Teslameter"=w356, "action"=enum16{"set", "get"}."set") -> ()  [unwired: 13 in, 1 out]
                  }
                }
                n252 = call <vilib>:"Release Semaphore.vi"("semaphore"=w72) -> ("semaphore out"=w71:T14)  [unwired: 5 in, 1 out]
                n253 = property on="Busy" class="Bool (strict)"(error in=w60, "Blinking"=FALSE) -> ()  [unwired: 1 in, 2 out]
              }
              frame True {
              }
            }
            n254 = Unbundle(w46) -> ("status"=w45:bool)  [unwired: 2 out]
            n255 = property on="error out" class="Clust (strict)"("Value"=w46, "Blinking"=w45) -> ()  [unwired: 2 in, 2 out]
            "loop 2" <- w51
          }
          n256 = call <vilib>:"Destroy Semaphore.vi"("semaphore"=w40) -> ()  [unwired: 5 in, 2 out]
          n257 = call "mergeError.vi"("error in (no error)"=w37, "error in (no error) 2"=w36) -> ("error out"=w39:errorcluster)  [unwired: 9 in]
        }
      }
    }
    frame Error {
    }
  }
  "VisaCluster" <- w3
  "error out" <- w1
